vi "angle process least distance.vi"(11 "Numeric in":dbl) -> (3 "Numeric out":dbl)   [LabVIEW 2019]
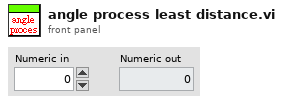
[diagram p1: front panel]
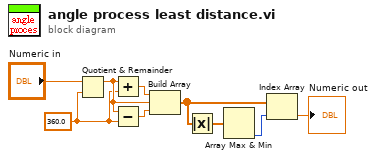
[diagram p0: block diagram]
diagram:
  w2 = 360.0 ("y")
  n1 = Quotient & Remainder(x="Numeric in", y=w2) -> (x-y*floor(x/y)=w5:dbl)  [unwired: 1 out]
  n2 = Add(x=w5, y=w2) -> (x+y=w4:dbl)
  n3 = Subtract(x=w5, y=w2) -> (x-y=w3:dbl)
  n4 = Build Array(w4, w5, w3) -> (w7:dbl[])
  n5 = Absolute Value(x=w7) -> (abs(x)=w6:dbl[])
  n6 = Array Max & Min(array=w6) -> (min index (indices)=w8:i32)  [unwired: 3 out]
  n7 = Index Array(array=w7, index=w8) -> (element=→"Numeric out":dbl)
